vi "Lifschitz-Kosevich function.vi"(10 "Temp":dbl[](array[numeric]), 11 "B (T)":dbl=14.69) -> (9 "Amp":dbl[](array[numeric]))   [LabVIEW 2020]
panel:
  in  "m*":dbl=14.69
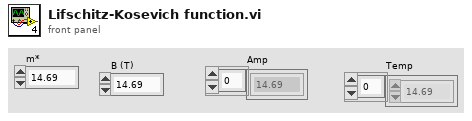
[diagram p1: front panel]
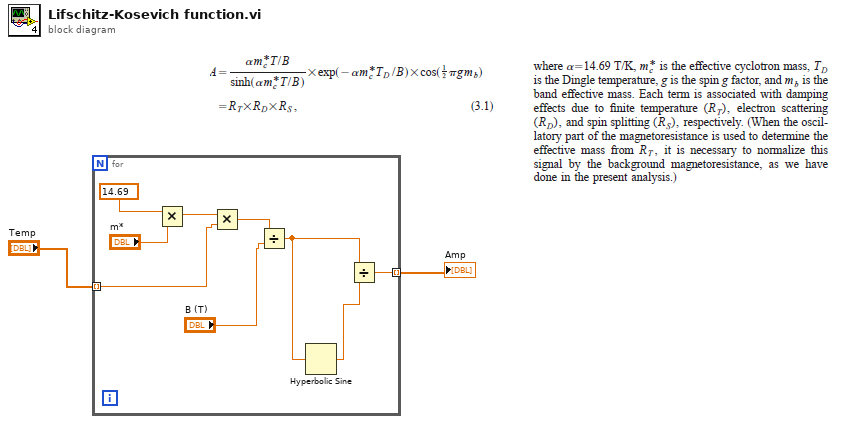
[diagram p0: block diagram]
diagram:
  n1 = for {
    tunnel: "Temp" -> [w5] mode=indexing
    tunnel: [w3] -> w1 mode=indexing
    n2 = Multiply(x=14.69, y="m*") -> (x*y=w9:dbl)
    n3 = Multiply(x=w9, y=w5) -> (x*y=w8:dbl)
    n4 = Divide(x=w8, y="B (T)") -> (x/y=w7:dbl)
    n5 = Hyperbolic Sine(1:w7) -> (0:w6:dbl)
    n6 = Divide(x=w7, y=w6) -> (x/y=w3:dbl)
  }
  "Amp" <- w1
